vi "NI6008 Status Report.vi"(8 "error in (no error)":errorcluster, 10 "Data":T1, 11 "Unit_Test_NI6008 in":refnum<class "Unit_Test_NI6008.lvclass">) -> (0 "error out":errorcluster, 3 "Unit_Test_NI6008 out":refnum<class "Unit_Test_NI6008.lvclass">)   [LabVIEW 2020, in "Unit_Test_NI6008.lvlib" / "Unit_Test_NI6008.lvclass"]
uses:
  Unit_Test_NI6008.lvclass
  Unit_Test_NI6008.lvclass/Unit_Test_NI6008.ctl
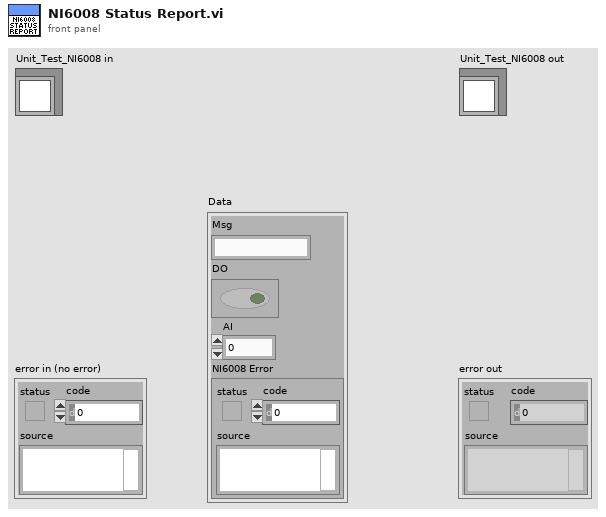
[diagram p1: front panel]
types:
  T1 = cluster{"Msg":string, "DO":bool[], "AI":dbl, "NI6008 Error":errorcluster}
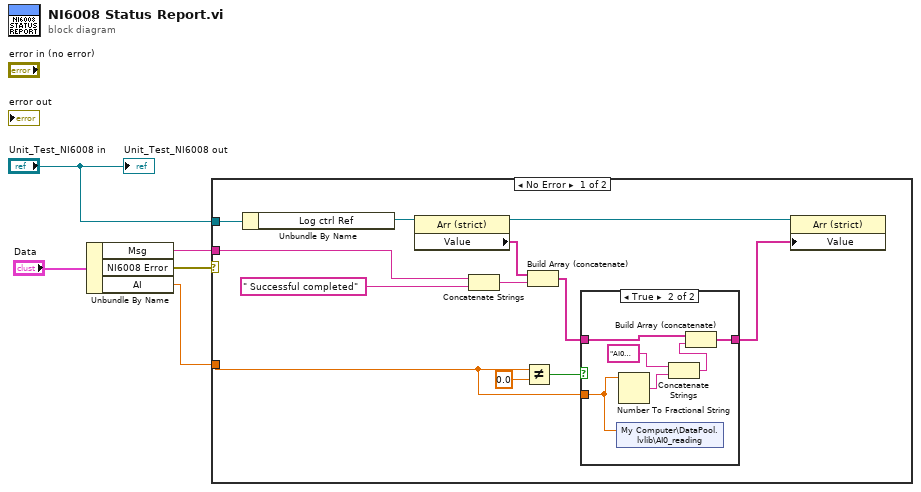
[diagram p0: block diagram]
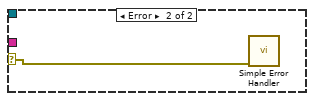
[diagram p3: hidden frame]
diagram:
  n1 = Unbundle By Name("Data") -> ("Msg"=w3:string, "NI6008 Error"=w4:errorcluster, "AI"=w1:dbl)
  n2 = case shown="No Error" w4 {
    selector: w4 -> [_ w25]
    tunnel: w3 -> [w13 _]
    tunnel: "Unit_Test_NI6008 in" -> [w17 _]
    tunnel: w1 -> [w7 _]
    frame No Error {
      n3 = Unbundle By Name(w17) -> ("Log ctrl Ref"=w16:refnum<vi>)
      n4 = property class="Arr (strict)"(reference=w16) -> (reference out=w15:refnum<vi>, "Value"=w14:string[])  [unwired: 1 in, 1 out]
      n5 = Concatenate Strings(w13, " Successful completed" ("string")) -> (w12:string)
      n6 = Not Equal?(x=w7, y=0.0) -> (x != y?=w9:bool)
      n7 = Build Array (concatenate)(w14, w12) -> (w8:string[])
      n8 = case shown="True" w9 {
        tunnel: w8 -> [w18 w24]
        tunnel: w7 -> [_ w19]
        tunnel: [w18 w20] -> w6
        frame False {
        }
        frame True {
          n9 = shared-variable "My Computer\\DataPool.lvlib\\AI0_reading"(w19) -> ()  [unwired: 1 in, 1 out]
          n10 = Number To Fractional String(number=w19) -> (F-format string=w21:string)  [unwired: 3 in]
          n11 = Concatenate Strings("AI0 Read Successful, reading is " ("string"), w21) -> (w23:string)
          n12 = Build Array (concatenate)(w24, w23) -> (w20:string[])
        }
      }
      n13 = property class="Arr (strict)"(reference=w15, "Value"=w6) -> ()  [unwired: 1 in, 2 out]
    }
    frame Error {
      n14 = call <vilib>:"Simple Error Handler.vi"("error in (no error)"=w25) -> ()  [unwired: 4 in, 5 out]
    }
  }
  "Unit_Test_NI6008 out" <- "Unit_Test_NI6008 in"
